vi "Check Data Size.vi"(8 "error in (no error)":errorcluster, 11 "UART Actor in":refnum<class "UART Actor.lvclass">) -> (0 "error out":errorcluster, 3 "UART Actor out":refnum<class "UART Actor.lvclass">)   [LabVIEW 2020, in "UART Actor.lvlib" / "UART Actor.lvclass"]
uses:
  UART Actor.lvclass
  UART Actor.lvclass/UART Actor.ctl
  <vilib>/ActorFramework/Time-Delayed Send Message/Time-Delay Override Options.ctl
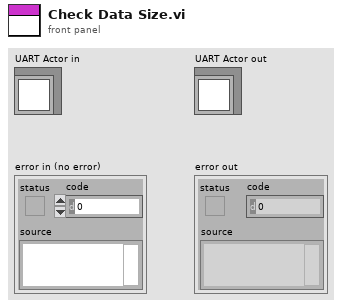
[diagram p1: front panel]
types:
  T1 = typedef "Time-Delay Override Options.ctl" = enum16{"Send next copy now", "Skip next scheduled copy", "Send next copy now and stop all further copies", "Stop all further copies"}
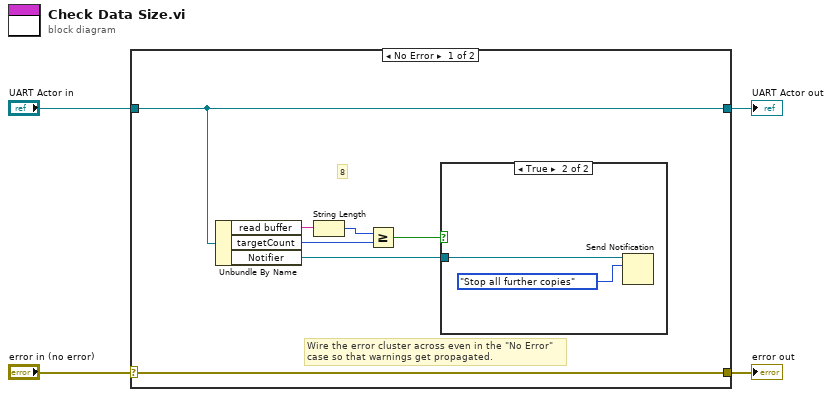
[diagram p0: block diagram]
diagram:
  n1 = case shown="No Error" "error in (no error)" {
    selector: "error in (no error)" -> [w11 w15]
    tunnel: [w11 w15] -> w3
    tunnel: [w9 w14] -> w1
    tunnel: "UART Actor in" -> [w9 w14]
    frame No Error {
      # "8"
      # "Wire the error cluster across even in the \"No Error\"\ncase so that warnings get propagated."
      n2 = Unbundle By Name(w9) -> ("read buffer"=w8:string, "targetCount"=w7:i32, "Notifier"=w5:refnum<notifier>)
      n3 = String Length(string=w8) -> (length=w10:i32)
      n4 = Greater Or Equal?(x=w10, y=w7) -> (x >= y?=w6:bool)
      n5 = case shown="True" w6 {
        tunnel: w5 -> [_ w13]
        frame False {
        }
        frame True {
          n6 = Send Notification(notification=Time-Delay_Override_Options."Stop all further copies", notifier=w13) -> ()  [unwired: 1 in, 2 out]
        }
      }
    }
    frame Error {
    }
  }
  "error out" <- w3
  "UART Actor out" <- w1
